vi "toAlim.vi"(8 "Error in":errorcluster, 9 "Entree":dbl, 11 "ID d'entrée":T1) -> (0 "Erreur en sortie":errorcluster caption="Error out", 3 "Device information out":string[](array[string]))   [LabVIEW 2019]
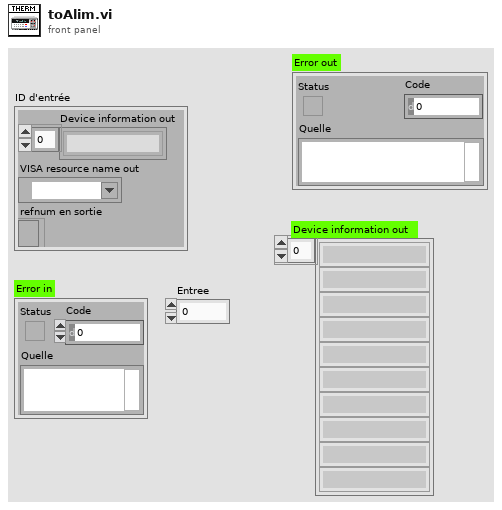
[diagram p1: front panel]
types:
  T1 = cluster{"Device information out":string[], "VISA resource name out":refnum<visa-resource-name>, "refnum en sortie":refnum<file>}
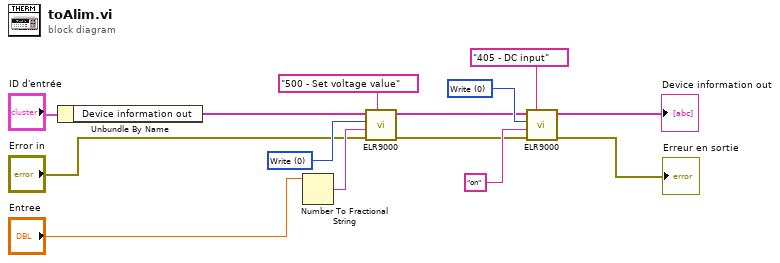
[diagram p0: block diagram]
diagram:
  w12 = u8 0 items=["Write", "Read"] ("Access")
  w14 = u8 0 items=["Write", "Read"] ("Access")
  n1 = Unbundle By Name("ID d'entrée") -> ("Device information out"=w4:string[])
  n2 = Number To Fractional String(number="Entree") -> (F-format string=w7:string)  [unwired: 3 in]
  n3 = call <instrlib>:"ELR9000.vi"("Command list"="500 - Set voltage value", "Error in"="Error in", "Value"=w7, "Access"=w14, "Device information in"=w4) -> ("Error out"=w9:errorcluster, "Device information out"=w10:string[])  [unwired: 1 in, 2 out]
  n4 = call <instrlib>:"ELR9000.vi"("Command list"="405 - DC input", "Error in"=w9, "Value"="on", "Access"=w12, "Device information in"=w10) -> ("Error out"=→"Erreur en sortie":errorcluster, "Device information out"=→"Device information out":string[])  [unwired: 1 in, 2 out]
